vi "(28) part 2 que.vi"() -> ()   [LabVIEW 2025]
panel:
  out "Numeric":i32
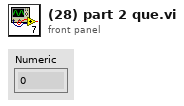
[diagram p1: front panel]
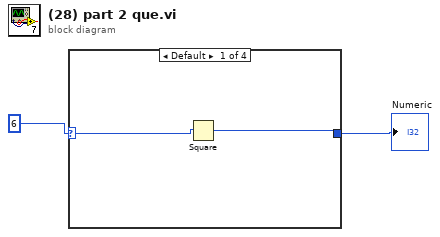
[diagram p0: block diagram]
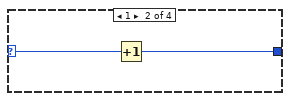
[diagram p2: hidden frame]
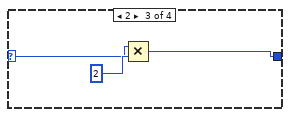
[diagram p3: hidden frame]
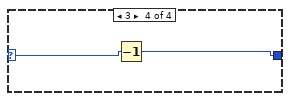
[diagram p4: hidden frame]
diagram:
  n1 = case shown="Default" 6 {
    selector: 6 -> [w4 w6 w8 w11]
    tunnel: [w3 w5 w7 w10] -> w1
    frame Default {
      n2 = Square(x=w4) -> (x^2=w3:i32)
    }
    frame 1 {
      n3 = Increment(x=w6) -> (x+1=w5:i32)
    }
    frame 2 {
      n4 = Multiply(x=w8, y=2) -> (x*y=w7:i32)
    }
    frame 3 {
      n5 = Decrement(x=w11) -> (x-1=w10:i32)
    }
  }
  "Numeric" <- w1
